vi "FormatMask.vi"(5 "mask":bool, 8 "encoded length":string) -> (2 "encoded length with mask":string)   [LabVIEW 2014, in "Raspberry Pi Compatible Compiler for LabVIEW.lvlib" / "Websocket.lvlib"]
uses:
  Websocket.lvlib
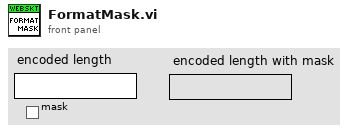
[diagram p1: front panel]
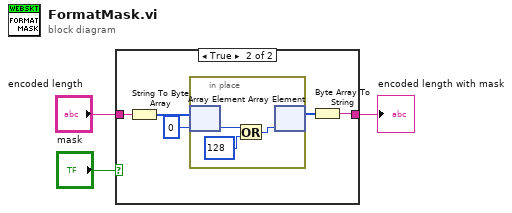
[diagram p0: block diagram]
diagram:
  n1 = case shown="True" "mask" {
    tunnel: "encoded length" -> [w4 w9]
    tunnel: [w4 w6] -> w1
    frame False {
    }
    frame True {
      n2 = String To Byte Array(string=w9) -> (unsigned byte array=w8:u8[])
      n3 = in-place {
        n4 = in-place-array #1(w8, 0) -> (w12:u8)
        n5 = Or(x=w12, y=u8 128) -> (x .or. y?=w11:u8)
        n6 = in-place-array #1(w11) -> (w5:u8[])  [unwired: 1 out]
      }
      n7 = Byte Array To String(unsigned byte array=w5) -> (string=w6:string)
    }
  }
  "encoded length with mask" <- w1
